vi "LASER.vi"(11 "State":i32) -> (1 "Fehler (Ausgang)":errorcluster, 3 "Speed":dbl)   [LabVIEW 2020]
uses:
  <vilib>/Instr/_visa.llb/VISA Configure Serial Port (Instr).vi
panel:
  out "IsState":i32
  out "Ausgabe String 2":string
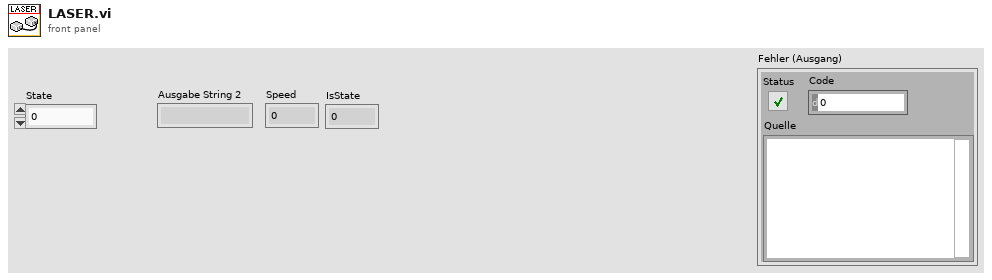
[diagram p1: front panel]
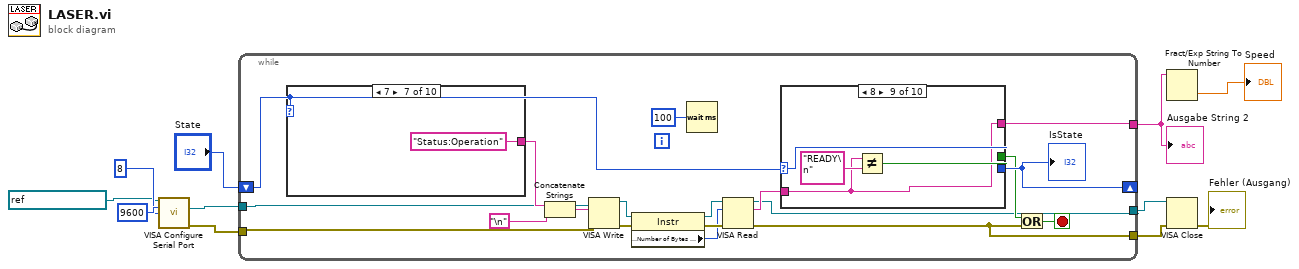
[diagram p0: block diagram]
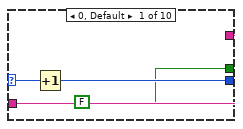
[diagram p2: hidden frame]
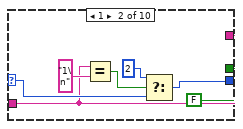
[diagram p3: hidden frame]
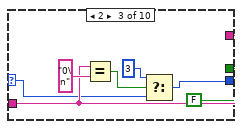
[diagram p4: hidden frame]
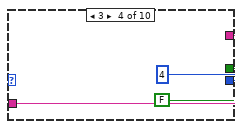
[diagram p5: hidden frame]
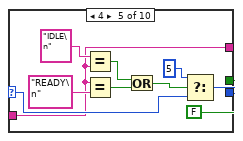
[diagram p6: hidden frame]
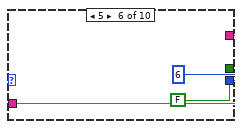
[diagram p7: hidden frame]
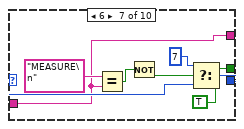
[diagram p8: hidden frame]
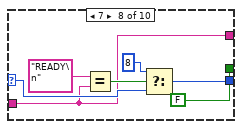
[diagram p9: hidden frame]
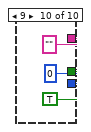
[diagram p10: hidden frame]
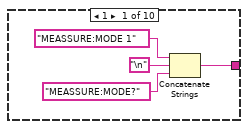
[diagram p11: hidden frame]
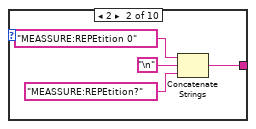
[diagram p12: hidden frame]
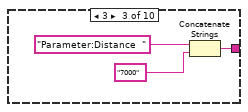
[diagram p13: hidden frame]
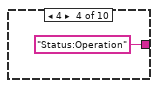
[diagram p14: hidden frame]
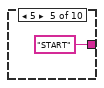
[diagram p15: hidden frame]
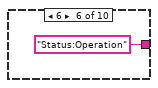
[diagram p16: hidden frame]
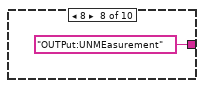
[diagram p17: hidden frame]
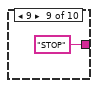
[diagram p18: hidden frame]
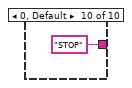
[diagram p19: hidden frame]
diagram:
  n1 = call-poly "VISA Configure Serial Port"("VISA resource name"=refnum<visa-resource-name> "ASRL1::INSTR", "baud rate (9600)"=u32 9600, "data bits (8)"=u16 8) -> ("VISA resource name out"=w1:refnum<visa-resource-name>, "error out"=w2:errorcluster)  [unwired: 11 in]
  n2 = while {
    shift-right: [w30] -> _
    shift-left: "State" -> [w28]
    tunnel: w2 -> [w19]
    tunnel: w1 -> [w17]
    tunnel: [w22] -> w4
    tunnel: [w13] -> w5
    tunnel: [w29] -> w6
    stop <- w12 stop-if-true
    n3 = case shown="7" w28 {
      tunnel: [w87 w91 w96 "Status:Operation" "START" "Status:Operation" "Status:Operation" "OUTPut:UNMEasurement" "STOP" "STOP"] -> w26
      frame 1 {
        n4 = Concatenate Strings("MEASSURE:MODE 1", "\n", "MEASSURE:MODE?") -> (w87:string)
      }
      frame 2 {
        n5 = Concatenate Strings("MEASSURE:REPEtition 0", "\n", "MEASSURE:REPEtition?") -> (w91:string)
      }
      frame 3 {
        n6 = Concatenate Strings("Parameter:Distance  ", "7000" ("String")) -> (w96:string)
      }
      frame 4 {
      }
      frame 5 {
      }
      frame 6 {
      }
      frame 7 {
      }
      frame 8 {
      }
      frame 9 {
      }
      frame 0, Default {
      }
    }
    n7 = Concatenate Strings(w26, "\n") -> (w18:string)
    n8 = VISA Write(VISA resource name=w17, write buffer=w18, error in (no error)=w19) -> (VISA resource name out=w15:refnum<visa-resource-name>, error out=w16:errorcluster)  [unwired: 1 out]
    n9 = property class="Instr"(reference=w15, error in=w16) -> (reference out=w20:refnum<visa-resource-name>, error out=w24:errorcluster, "Serial Settings:Number of Bytes at Serial Port"=w21:u32)
    n10 = Wait (ms)(milliseconds to wait=u32 100 ("Zu wartende ms")) -> ()  [unwired: 1 out]
    n11 = VISA Read(VISA resource name=w20, byte count=w21, error in (no error)=w24) -> (VISA resource name out=w22:refnum<visa-resource-name>, read buffer=w23:string, error out=w13:errorcluster)  [unwired: 1 out]
    n12 = case "Case-Struktur" shown="8" w28 {
      selector: w28 -> [w33 w37 w43 _ w54 _ w71 w76 w83 _]
      tunnel: [w32 w38 w44 4 ("State") w55 6 ("State") w70 w75 w83 0 ("State")] -> w30
      tunnel: w23 -> [w34 w36 w45 w51 w53 w63 w69 w74 w80 _]
      tunnel: [w34 w36 w45 w51 w53 w63 w69 w74 w80 "" ("read buffer")] -> w29
      tunnel: [FALSE FALSE FALSE FALSE FALSE FALSE TRUE FALSE w82 TRUE] -> w27
      frame 0, Default {
        n13 = Increment(x=w33) -> (x+1=w32:i32)
      }
      frame 1 {
        n14 = Equal?(x=w36, y="1\n") -> (x = y?=w41:bool)
        n15 = Select(t=2, s=w41, f=w37) -> (s? t:f=w38:i32)
      }
      frame 2 {
        n16 = Equal?(x=w45, y="0\n") -> (x = y?=w48:bool)
        n17 = Select(t=3, s=w48, f=w43) -> (s? t:f=w44:i32)
      }
      frame 3 {
      }
      frame 4 {
        n18 = Equal?(x="IDLE\n", y=w53) -> (x = y?=w61:bool)
        n19 = Equal?(x=w53, y="READY\n") -> (x = y?=w60:bool)
        n20 = Or(x=w61, y=w60) -> (x .or. y?=w58:bool)
        n21 = Select(t=5, s=w58, f=w54) -> (s? t:f=w55:i32)
      }
      frame 5 {
      }
      frame 6 {
        n22 = Equal?(x="MEASURE\n", y=w69) -> (x = y?=w67:bool)
        n23 = Not(x=w67) -> (.not. x?=w66:bool)
        n24 = Select(t=7, s=w66, f=w71) -> (s? t:f=w70:i32)
      }
      frame 7 {
        n25 = Equal?(x="READY\n", y=w74) -> (x = y?=w77:bool)
        n26 = Select(t=8, s=w77, f=w76) -> (s? t:f=w75:i32)
      }
      frame 8 {
        n27 = Not Equal?(x=w80, y="READY\n" ("x")) -> (x != y?=w82:bool)
      }
      frame 9 {
      }
    }
    "IsState" <- w30
    n28 = Or(x=w27, y=w13) -> (x .or. y?=w12:bool)
  }
  "Ausgabe String 2" <- w6
  n29 = Fract/Exp String To Number(string=w6) -> (number=→"Speed":dbl)  [unwired: 3 in, 1 out]
  n30 = VISA Close(VISA resource name=w4, error in (no error)=w5) -> (error out=→"Fehler (Ausgang)":errorcluster)
